vi "visaWrite.vi"(8 "Error in":errorcluster, 11 "VISA in":refnum<visa-resource-name>) -> (0 "Error out":errorcluster, 3 "VISA out":refnum<visa-resource-name>)   [LabVIEW 2014, in "libMux.lvlib"]
uses:
  libMux.lvlib
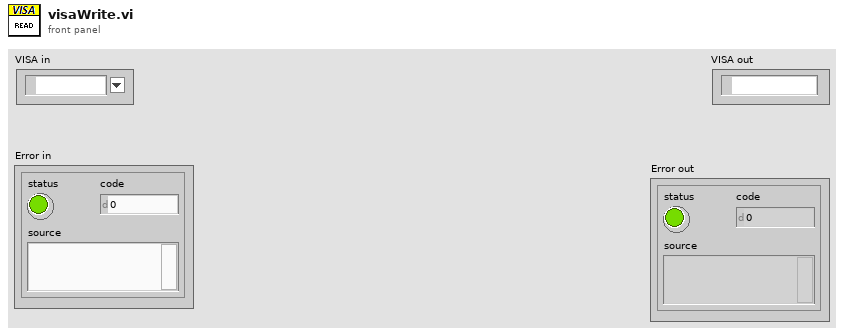
[diagram p1: front panel]
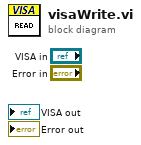
[diagram p0: block diagram]
diagram:
